vi "Lockin Control Panel.vi"() -> ()   [LabVIEW 2021]
uses:
  <instrlib>/Stanford Research 830/Public/Data/Read (All Parameters).vi
  <instrlib>/Stanford Research 830/Stanford Research 830.lvlib
panel:
  in  "Display 2 Sel":u16(ring)=1 items=["X", "Y", "R", "Theta", "Aux In 1", "Aux In 2", "Aux In 3", "Aux In 4", "Ref Freq", "Ch1 Disp", "Ch2 Disp"]
  in  "Display 1 Sel":u16(ring)=1 items=["X", "Y", "R", "Theta", "Aux In 1", "Aux In 2", "Aux In 3", "Aux In 4", "Ref Freq", "Ch1 Disp", "Ch2 Disp"]
  out "Display 2":dbl format="%.3p"
  in  "Update":bool
  out "Display 1":dbl format="%.3p"
  in  "Reset":bool
  in  "Init":bool
  in  "Set Input":bool
  in  "Float/GND":bool
  in  "AC/DC":bool
  in  "Input":u16(ring) items=["A", "A-B", "I (1MOhm", "I (100MOhm"]
  in  "Refresh":bool
  in  "Auto Phase":bool
  in  "Set Ref":bool
  in  "Phase":dbl
  in  "Reference Source":u16(ring) items=["External", "Internal"]
  in  "Time Constant":u16(ring) items=["10 us", "30 us", "100 us", "300 us", "1 ms", "3 ms", "10 ms", "30 ms", "100 ms", "300 ms", "1 s", "3 s", "10 s", "30 s", "100 s", "300 s", "1 ks", "3 ks", "10 ks", "30 ks"]
  in  "Set TC and SEN":bool
  in  "Sensitivity":i16(ring)=-1 items=["2 nV/fA", "5 nV/fA", "10 nV/fA", "20 nV/fA", "50 nV/fA", "100 nV/fA", "200 nV/fA", "500 nV/fA", "1 uV/pA", "2 uV/pA", "5 uV/pA", "10 uV/pA", "20 uV/pA", "50 uV/pA", "100 uV/pA", "200 uV/pA", "500 uV/pA", "1 mV/nA", "2 mV/nA", "5 mV/nA", "10 mV/nA", "20 mV/nA", "50 mV/nA", "100 mV/nA", "200 mV/nA", "500 mV/nA", "1 V/uA"]
  in  "Quit":bool
  in  "Set OSC":bool
  in  "Amplitude":dbl format="%.6f V"
  in  "Frequency":dbl format="%.3f Hz"
  in  "Connect":bool
  in  "Model":enum16{"7265", "SR830"}(ring)=enum."SR830"
  in  "VISA resource name":refnum<visa-resource-name>
  # "Input"
  # "Measure"
  # "Reference"
  # "Oscillator"
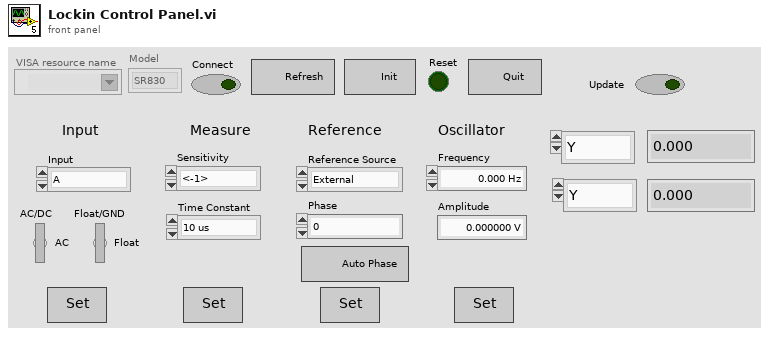
[diagram p1: front panel]
types:
  T1 = enum8{"Enabled", "Disabled", "Disabled and Grayed Out"}
  T2 = cluster{"X-Value":dbl, "Y-Value":dbl, "R-Value":dbl, "Theta-Value":dbl, "Aux In 1 Value":dbl, "Aux In 2 Value":dbl, "Aux In 3 Value":dbl, "Aux In 4 Value":dbl, "Reference Frequency":dbl, "Channel 1 Display":dbl, "Channel 2 Display":dbl}
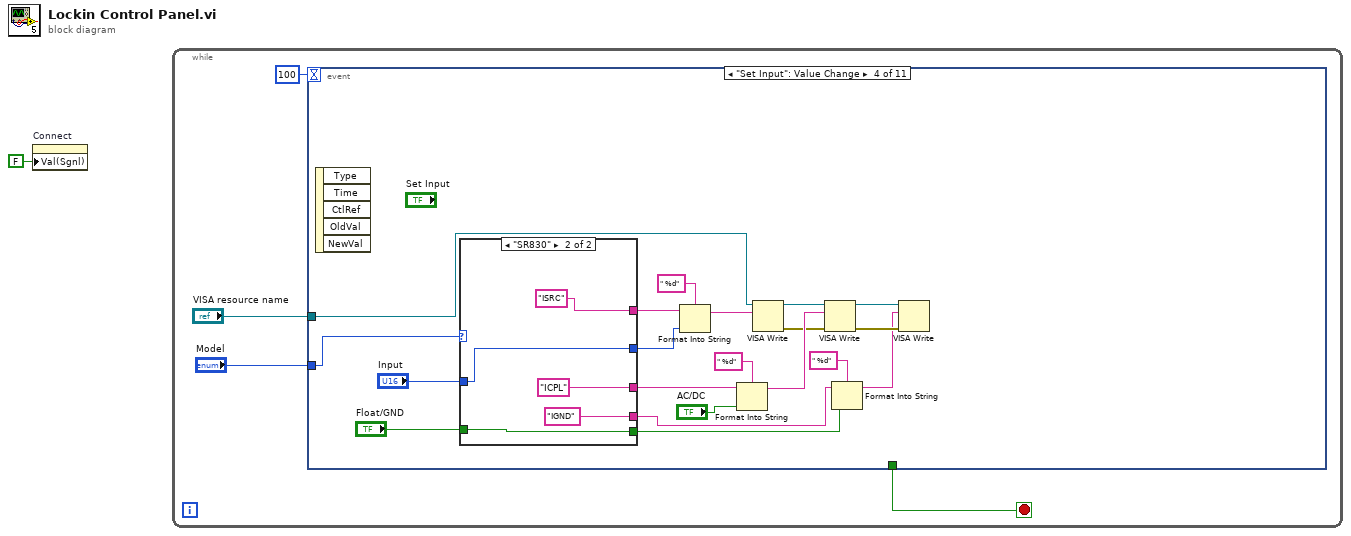
[diagram p0: block diagram]
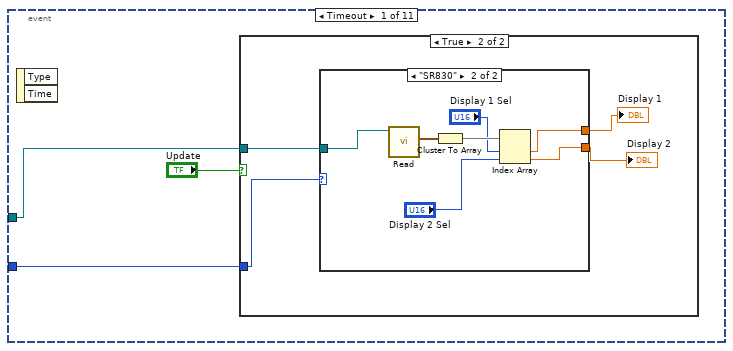
[diagram p2: hidden frame]
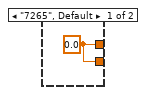
[diagram p4: hidden frame]
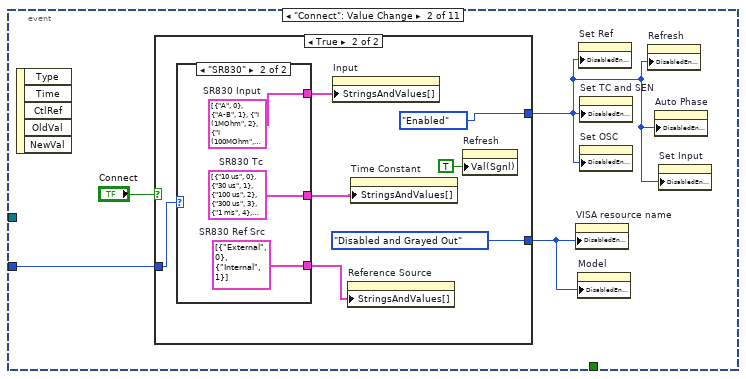
[diagram p5: hidden frame]
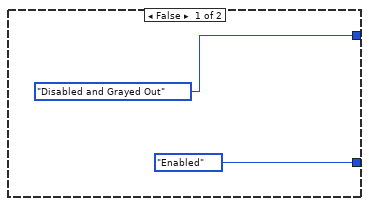
[diagram p6: hidden frame]
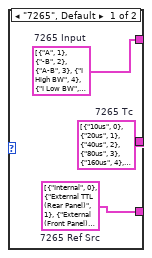
[diagram p7: hidden frame]
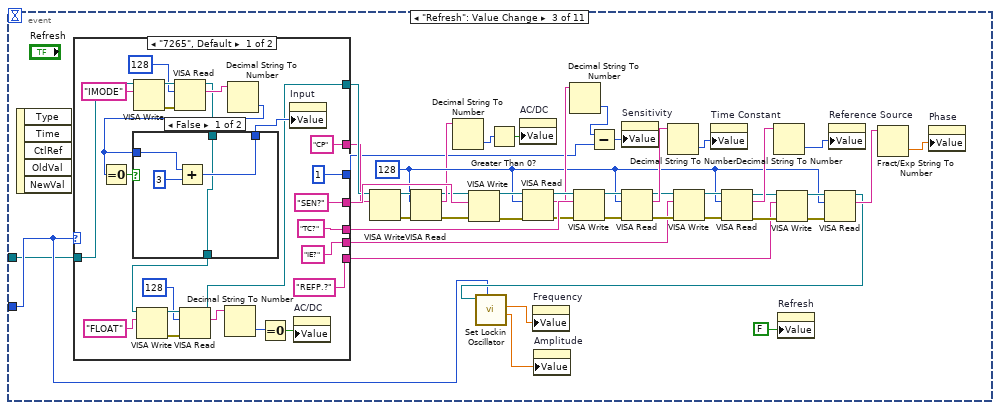
[diagram p8: hidden frame]
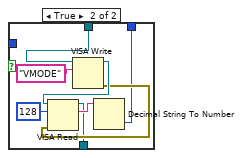
[diagram p9: hidden frame]
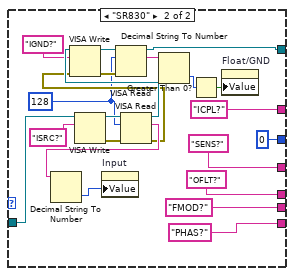
[diagram p10: hidden frame]
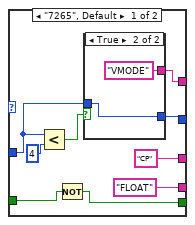
[diagram p11: hidden frame]
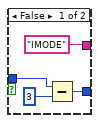
[diagram p12: hidden frame]
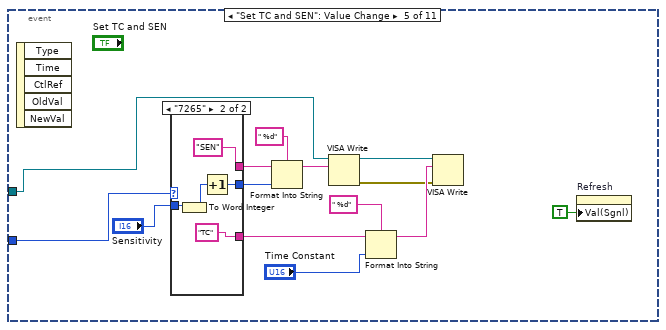
[diagram p13: hidden frame]
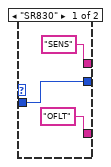
[diagram p14: hidden frame]
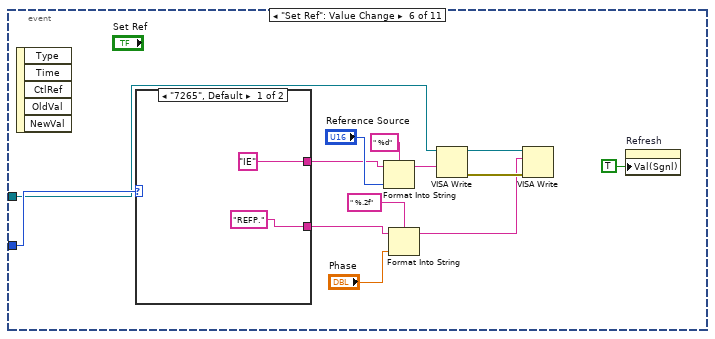
[diagram p15: hidden frame]
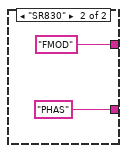
[diagram p16: hidden frame]
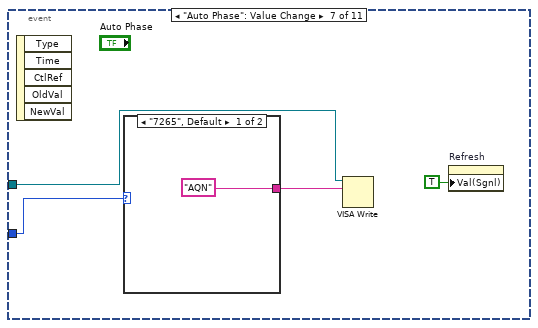
[diagram p17: hidden frame]
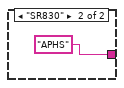
[diagram p18: hidden frame]
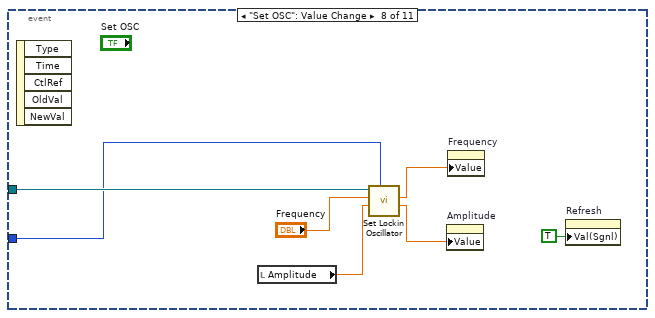
[diagram p19: hidden frame]
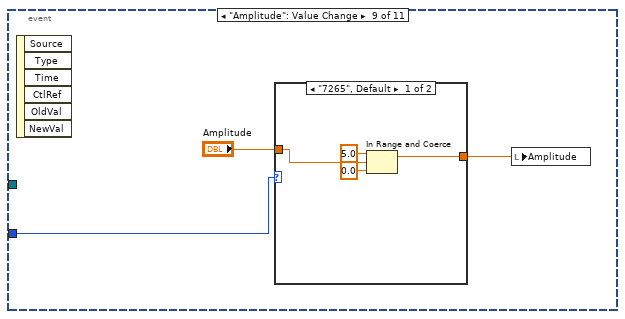
[diagram p20: hidden frame]
diagram:
  n1 = property on="Connect" class="Bool (strict)"("Val(Sgnl)"=FALSE ("Value (Signaling)")) -> ()  [unwired: 2 in, 2 out]
  n2 = while {
    stop <- w5 stop-if-true
    n3 = event shown="[3] \"Set Input\": Value Change" {
      selector: _ -> [_ _ _ _ _ _ _ _ _ _ _]
      dyn-events: _ -> [_ _ _ _ _ _ _ _ _ _ _]
      timeout: 100 -> [_ _ _ _ _ _ _ _ _ _ _]
      tunnel: [_ _ _ _ _ _ _ _ _ _ "Quit"] -> w5
      tunnel: "VISA resource name" -> [w7 _ w50 w156 w196 w213 w223 w234 _ w246 _]
      tunnel: "Model" -> [w6 w23 w58 w162 w195 w217 w225 w233 w237 w247 _]
      event Timeout {
        n4 = event-data() -> ()  [unwired: 1 in, 2 out]
        n5 = case shown="True" "Update" {
          tunnel: w7 -> [_ w12]
          tunnel: w6 -> [_ w11]
          frame False {
          }
          frame True {
            n6 = case shown="\"SR830\"" w11 {
              tunnel: w12 -> [_ w20]
              tunnel: [w13 w16] -> w10
              tunnel: [w13 w15] -> w9
              frame "7265", Default {
                w13 = 0.0 ("X-Value")
              }
              frame "SR830" {
                n7 = call-poly <instrlib>:"Read.vi"("VISA resource name"=w20) -> ("Parameter Values"=w19:T2)  [unwired: 8 in, 2 out]
                n8 = Cluster To Array(cluster=w19) -> (array=w18:dbl[])
                n9 = Index Array(array=w18, index #1="Display 1 Sel", index #2="Display 2 Sel") -> (element #1=w16:dbl, element #2=w15:dbl)
              }
            }
            "Display 1" <- w10
            "Display 2" <- w9
          }
        }
      }
      event "Connect": Value Change {
        n10 = event-data() -> ()  [unwired: 1 in, 5 out]
        n11 = case shown="True" "Connect" {
          tunnel: w23 -> [_ w33]
          tunnel: [T1."Enabled" ("Disabled") T1."Disabled and Grayed Out" ("Disabled")] -> w22
          tunnel: [T1."Disabled and Grayed Out" ("Disabled") T1."Enabled" ("Disabled")] -> w21
          frame False {
          }
          frame True {
            n12 = case shown="\"SR830\"" w33 {
              tunnel: [w36 w39] -> w32
              tunnel: [w35 w38] -> w29
              tunnel: [w34 w37] -> w27
              frame "7265", Default {
                w34 = cluster{"String":string, "Value":u16}[] [{"String"="A", "Value"=1}, {"String"="-B", "Value"=2}, {"String"="A-B", "Value"=3}, {"String"="I High BW", "Value"=4}, {"String"="I Low BW", "Value"=5}]  # 7265 Input
                w35 = cluster{"String":string, "Value":u8}[] [{"String"="Internal", "Value"=0}, {"String"="External TTL (Rear Panel)", "Value"=1}, {"String"="External (Front Panel)", "Value"=2}]  # 7265 Ref Src
                w36 = cluster{"String":string, "Value":u16}[] [{"String"="10us", "Value"=0}, {"String"="20us", "Value"=1}, {"String"="40us", "Value"=2}, {"String"="80us", "Value"=3}, {"String"="160us", "Value"=4}, {"String"="320us", "Value"=5}, {"String"="640us", "Value"=6}, {"String"="5ms", "Value"=7}, {"String"="10ms", "Value"=8}, {"String"="20ms", "Value"=9}, {"String"="50ms", "Value"=10}, {"String"="100ms", "Value"=11}, {"String"="200ms", "Value"=12}, {"String"="500ms", "Value"=13}, {"String"="1s", "Value"=14}, {"String"="2s", "Value"=15}, {"String"="5s", "Value"=16}, {"String"="10s", "Value"=17}, {"String"="20s", "Value"=18}, {"String"="50s", "Value"=19}, {"String"="100s", "Value"=20}, {"String"="200s", "Value"=21}, {"String"="500s", "Value"=22}, {"String"="1ks", "Value"=23}, {"String"="2ks", "Value"=24}, {"String"="5ks", "Value"=25}, {"String"="10ks", "Value"=26}, {"String"="20ks", "Value"=27}, {"String"="50ks", "Value"=28}, {"String"="100ks", "Value"=29}]  # 7265 Tc
              }
              frame "SR830" {
                w37 = cluster{"String":string, "Value":u16}[] [{"String"="A", "Value"=0}, {"String"="A-B", "Value"=1}, {"String"="I (1MOhm", "Value"=2}, {"String"="I (100MOhm", "Value"=3}]  # SR830 Input
                w38 = cluster{"String":string, "Value":u16}[] [{"String"="External", "Value"=0}, {"String"="Internal", "Value"=1}]  # SR830 Ref Src
                w39 = cluster{"String":string, "Value":u16}[] [{"String"="10 us", "Value"=0}, {"String"="30 us", "Value"=1}, {"String"="100 us", "Value"=2}, {"String"="300 us", "Value"=3}, {"String"="1 ms", "Value"=4}, {"String"="3 ms", "Value"=5}, {"String"="10 ms", "Value"=6}, {"String"="30 ms", "Value"=7}, {"String"="100 ms", "Value"=8}, {"String"="300 ms", "Value"=9}, {"String"="1 s", "Value"=10}, {"String"="3 s", "Value"=11}, {"String"="10 s", "Value"=12}, {"String"="30 s", "Value"=13}, {"String"="100 s", "Value"=14}, {"String"="300 s", "Value"=15}, {"String"="1 ks", "Value"=16}, {"String"="3 ks", "Value"=17}, {"String"="10 ks", "Value"=18}, {"String"="30 ks", "Value"=19}]  # SR830 Tc
              }
            }
            n13 = property on="Input" class="Ring (strict)"("StringsAndValues[]"=w27) -> ()  [unwired: 2 in, 2 out]
            n14 = property on="Reference Source" class="Ring (strict)"("StringsAndValues[]"=w29) -> ()  [unwired: 2 in, 2 out]
            n15 = property on="Time Constant" class="Ring (strict)"("StringsAndValues[]"=w32) -> ()  [unwired: 2 in, 2 out]
            n16 = property on="Refresh" class="Bool (strict)"("Val(Sgnl)"=TRUE ("Value (Signaling)")) -> ()  [unwired: 2 in, 2 out]
          }
        }
        n17 = property on="VISA resource name" class="VISAName"("DisabledEnum"=w22) -> ()  [unwired: 2 in, 2 out]
        n18 = property on="Model" class="Enum (strict)"("DisabledEnum"=w22) -> ()  [unwired: 2 in, 2 out]
        n19 = property on="Set Ref" class="Bool"("DisabledEnum"=w21) -> ()  [unwired: 2 in, 2 out]
        n20 = property on="Set TC and SEN" class="Bool"("DisabledEnum"=w21) -> ()  [unwired: 2 in, 2 out]
        n21 = property on="Set OSC" class="Bool"("DisabledEnum"=w21) -> ()  [unwired: 2 in, 2 out]
        n22 = property on="Refresh" class="Bool (strict)"("DisabledEnum"=w21) -> ()  [unwired: 2 in, 2 out]
        n23 = property on="Auto Phase" class="Bool"("DisabledEnum"=w21) -> ()  [unwired: 2 in, 2 out]
        n24 = property on="Set Input" class="Bool"("DisabledEnum"=w21) -> ()  [unwired: 2 in, 2 out]
      }
      event "Refresh": Value Change {
        w48 = u32 128 ("byte count")
        n25 = event-data() -> ()  [unwired: 1 in, 5 out]
        n26 = case shown="\"7265\", Default" w58 {
          tunnel: ["SEN?" "SENS?"] -> w49
          tunnel: ["TC?" "OFLT?"] -> w81
          tunnel: ["IE?" "FMOD?"] -> w69
          tunnel: ["REFP.?" "PHAS?"] -> w62
          tunnel: ["CP" "ICPL?"] -> w43
          tunnel: w50 -> [w103 w134]
          tunnel: [w87 w123] -> w46
          tunnel: [1 0] -> w40
          frame "7265", Default {
            n27 = VISA Write(VISA resource name=w103, write buffer="IMODE") -> (VISA resource name out=w102:refnum<visa-resource-name>, error out=w100:errorcluster)  [unwired: 1 in, 1 out]
            n28 = VISA Read(VISA resource name=w102, byte count=128, error in (no error)=w100) -> (VISA resource name out=w95:refnum<visa-resource-name>, read buffer=w98:string)  [unwired: 2 out]
            n29 = Decimal String To Number(string=w98) -> (number=w96:i32)  [unwired: 2 in, 1 out]
            n30 = Equal To 0?(x=w96) -> (x = 0?=w97:bool)
            n31 = case shown="False" w97 {
              tunnel: w96 -> [w112 _]
              tunnel: w95 -> [w109 w120]
              tunnel: [w110 w114] -> w94
              tunnel: [w109 w113] -> w92
              frame False {
                n32 = Add(x=w112, y=3) -> (x+y=w110:i32)
              }
              frame True {
                n33 = VISA Write(VISA resource name=w120, write buffer="VMODE") -> (VISA resource name out=w118:refnum<visa-resource-name>, error out=w117:errorcluster)  [unwired: 1 in, 1 out]
                n34 = VISA Read(VISA resource name=w118, byte count=u32 128, error in (no error)=w117) -> (VISA resource name out=w113:refnum<visa-resource-name>, read buffer=w115:string)  [unwired: 2 out]
                n35 = Decimal String To Number(string=w115) -> (number=w114:i32)  [unwired: 2 in, 1 out]
              }
            }
            n36 = VISA Write(VISA resource name=w92, write buffer="FLOAT") -> (VISA resource name out=w91:refnum<visa-resource-name>, error out=w89:errorcluster)  [unwired: 1 in, 1 out]
            n37 = VISA Read(VISA resource name=w91, byte count=u32 128, error in (no error)=w89) -> (VISA resource name out=w87:refnum<visa-resource-name>, read buffer=w88:string)  [unwired: 2 out]
            n38 = Decimal String To Number(string=w88) -> (number=w86:i32)  [unwired: 2 in, 1 out]
            n39 = Equal To 0?(x=w86) -> (x = 0?=w85:bool)
            n40 = property on="Input" class="Ring (strict)"("Value"=w94) -> ()  [unwired: 2 in, 2 out]
            n41 = property on="AC/DC" class="Bool (strict)"("Value"=w85) -> ()  [unwired: 2 in, 2 out]
          }
          frame "SR830" {
            w122 = u32 128 ("byte count")
            n42 = VISA Write(VISA resource name=w134, write buffer="ISRC?") -> (VISA resource name out=w137:refnum<visa-resource-name>, error out=w136:errorcluster)  [unwired: 1 in, 1 out]
            n43 = VISA Read(VISA resource name=w137, byte count=w122, error in (no error)=w136) -> (VISA resource name out=w130:refnum<visa-resource-name>, read buffer=w132:string, error out=w129:errorcluster)  [unwired: 1 out]
            n44 = Decimal String To Number(string=w132) -> (number=w133:i32)  [unwired: 2 in, 1 out]
            n45 = VISA Write(VISA resource name=w130, write buffer="IGND?", error in (no error)=w129) -> (VISA resource name out=w131:refnum<visa-resource-name>, error out=w128:errorcluster)  [unwired: 1 out]
            n46 = property on="Input" class="Ring (strict)"("Value"=w133) -> ()  [unwired: 2 in, 2 out]
            n47 = VISA Read(VISA resource name=w131, byte count=w122, error in (no error)=w128) -> (VISA resource name out=w123:refnum<visa-resource-name>, read buffer=w124:string)  [unwired: 2 out]
            n48 = Decimal String To Number(string=w124) -> (number=w126:i32)  [unwired: 2 in, 1 out]
            n49 = Greater Than 0?(x=w126) -> (x > 0?=w125:bool)
            n50 = property on="Float/GND" class="Bool (strict)"("Value"=w125) -> ()  [unwired: 2 in, 2 out]
          }
        }
        n51 = VISA Write(VISA resource name=w46, write buffer=w43) -> (VISA resource name out=w53:refnum<visa-resource-name>, error out=w54:errorcluster)  [unwired: 1 in, 1 out]
        n52 = VISA Read(VISA resource name=w53, byte count=w48, error in (no error)=w54) -> (VISA resource name out=w44:refnum<visa-resource-name>, read buffer=w47:string, error out=w45:errorcluster)  [unwired: 1 out]
        n53 = Decimal String To Number(string=w47) -> (number=w52:i32)  [unwired: 2 in, 1 out]
        n54 = VISA Write(VISA resource name=w44, write buffer=w49, error in (no error)=w45) -> (VISA resource name out=w83:refnum<visa-resource-name>, error out=w82:errorcluster)  [unwired: 1 out]
        n55 = Greater Than 0?(x=w52) -> (x > 0?=w51:bool)
        n56 = property on="AC/DC" class="Bool (strict)"("Value"=w51) -> ()  [unwired: 2 in, 2 out]
        n57 = VISA Read(VISA resource name=w83, byte count=w48, error in (no error)=w82) -> (VISA resource name out=w79:refnum<visa-resource-name>, read buffer=w78:string, error out=w80:errorcluster)  [unwired: 1 out]
        n58 = Decimal String To Number(string=w78) -> (number=w42:i32)  [unwired: 2 in, 1 out]
        n59 = VISA Write(VISA resource name=w79, write buffer=w81, error in (no error)=w80) -> (VISA resource name out=w77:refnum<visa-resource-name>, error out=w76:errorcluster)  [unwired: 1 out]
        n60 = Subtract(x=w42, y=w40) -> (x-y=w41:i32)
        n61 = property on="Sensitivity" class="Ring (strict)"("Value"=w41) -> ()  [unwired: 2 in, 2 out]
        n62 = VISA Read(VISA resource name=w77, byte count=w48, error in (no error)=w76) -> (VISA resource name out=w71:refnum<visa-resource-name>, read buffer=w74:string, error out=w70:errorcluster)  [unwired: 1 out]
        n63 = Decimal String To Number(string=w74) -> (number=w75:i32)  [unwired: 2 in, 1 out]
        n64 = VISA Write(VISA resource name=w71, write buffer=w69, error in (no error)=w70) -> (VISA resource name out=w73:refnum<visa-resource-name>, error out=w72:errorcluster)  [unwired: 1 out]
        n65 = property on="Time Constant" class="Ring (strict)"("Value"=w75) -> ()  [unwired: 2 in, 2 out]
        n66 = VISA Read(VISA resource name=w73, byte count=w48, error in (no error)=w72) -> (VISA resource name out=w64:refnum<visa-resource-name>, read buffer=w67:string, error out=w63:errorcluster)  [unwired: 1 out]
        n67 = Decimal String To Number(string=w67) -> (number=w68:i32)  [unwired: 2 in, 1 out]
        n68 = VISA Write(VISA resource name=w64, write buffer=w62, error in (no error)=w63) -> (VISA resource name out=w66:refnum<visa-resource-name>, error out=w65:errorcluster)  [unwired: 1 out]
        n69 = property on="Refresh" class="Bool (strict)"("Value"=FALSE ("Refresh")) -> ()  [unwired: 2 in, 2 out]
        n70 = VISA Read(VISA resource name=w66, byte count=w48, error in (no error)=w65) -> (VISA resource name out=w59:refnum<visa-resource-name>, read buffer=w60:string)  [unwired: 2 out]
        n71 = call "Set Lockin Oscillator.vi"("Model"=w58, "VISA resource name"=w59) -> ("Actual Amp"=w56:dbl, "Actual Freq"=w57:dbl)  [unwired: 8 in]
        n72 = property on="Frequency" class="DigNum (strict)"("Value"=w57) -> ()  [unwired: 2 in, 2 out]
        n73 = property on="Amplitude" class="DigNum (strict)"("Value"=w56) -> ()  [unwired: 2 in, 2 out]
        n74 = property on="Reference Source" class="Ring (strict)"("Value"=w68) -> ()  [unwired: 2 in, 2 out]
        n75 = Fract/Exp String To Number(string=w60) -> (number=w61:dbl)  [unwired: 3 in, 1 out]
        n76 = property on="Phase" class="DigNum (strict)"("Value"=w61) -> ()  [unwired: 2 in, 2 out]
      }
      event "Set Input": Value Change {
        n77 = event-data() -> ()  [unwired: 1 in, 5 out]
        n78 = case shown="\"SR830\"" w162 {
          tunnel: "Input" -> [w167 w182]
          tunnel: [w168 w182] -> w160
          tunnel: [w169 "ISRC"] -> w159
          tunnel: ["CP" "ICPL"] -> w153
          tunnel: ["FLOAT" "IGND"] -> w146
          tunnel: "Float/GND" -> [w164 w178]
          tunnel: [w163 w178] -> w144
          frame "7265", Default {
            n79 = Less?(x=w167, y=u16 4) -> (x < y?=w170:bool)
            n80 = Not(x=w164) -> (.not. x?=w163:bool)
            n81 = case shown="True" w170 {
              tunnel: ["IMODE" "VMODE"] -> w169
              tunnel: [w174 w176] -> w168
              tunnel: w167 -> [w173 w176]
              frame False {
                n82 = Subtract(x=w173, y=u16 3) -> (x-y=w174:u16)
              }
              frame True {
              }
            }
          }
          frame "SR830" {
          }
        }
        n83 = Format Into String(format string=" %d", initial string=w159, w160) -> (resulting string=w157:string)  [unwired: 1 in, 1 out]
        n84 = Format Into String(format string=" %d", initial string=w153, "AC/DC") -> (resulting string=w151:string)  [unwired: 1 in, 1 out]
        n85 = VISA Write(VISA resource name=w156, write buffer=w157) -> (VISA resource name out=w150:refnum<visa-resource-name>, error out=w149:errorcluster)  [unwired: 1 in, 1 out]
        n86 = VISA Write(VISA resource name=w150, write buffer=w151, error in (no error)=w149) -> (VISA resource name out=w147:refnum<visa-resource-name>, error out=w148:errorcluster)  [unwired: 1 out]
        n87 = Format Into String(format string=" %d", initial string=w146, w144) -> (resulting string=w143:string)  [unwired: 1 in, 1 out]
        n88 = VISA Write(VISA resource name=w147, write buffer=w143, error in (no error)=w148) -> ()  [unwired: 3 out]
      }
      event "Set TC and SEN": Value Change {
        n89 = event-data() -> ()  [unwired: 1 in, 5 out]
        n90 = case shown="\"7265\"" w195 {
          tunnel: ["SENS" "SEN"] -> w194
          tunnel: "Sensitivity" -> [w198 w202]
          tunnel: [w198 w203] -> w191
          tunnel: ["OFLT" "TC"] -> w189
          frame "SR830" {
          }
          frame "7265" {
            n91 = To Word Integer(number=w202) -> (16bit integer=w201:i16)
            n92 = Increment(x=w201) -> (x+1=w203:i16)
          }
        }
        n93 = Format Into String(format string=" %d", initial string=w194, w191) -> (resulting string=w190:string)  [unwired: 1 in, 1 out]
        n94 = VISA Write(VISA resource name=w196, write buffer=w190) -> (VISA resource name out=w186:refnum<visa-resource-name>, error out=w184:errorcluster)  [unwired: 1 in, 1 out]
        n95 = Format Into String(format string=" %d", initial string=w189, "Time Constant") -> (resulting string=w185:string)  [unwired: 1 in, 1 out]
        n96 = VISA Write(VISA resource name=w186, write buffer=w185, error in (no error)=w184) -> ()  [unwired: 3 out]
        n97 = property on="Refresh" class="Bool (strict)"("Val(Sgnl)"=TRUE ("Value (Signaling)")) -> ()  [unwired: 2 in, 2 out]
      }
      event "Set Ref": Value Change {
        n98 = event-data() -> ()  [unwired: 1 in, 5 out]
        n99 = case shown="\"7265\", Default" w217 {
          tunnel: ["IE" "FMOD"] -> w215
          tunnel: ["REFP." "PHAS"] -> w211
          frame "7265", Default {
          }
          frame "SR830" {
          }
        }
        n100 = Format Into String(format string=" %d", initial string=w215, "Reference Source") -> (resulting string=w212:string)  [unwired: 1 in, 1 out]
        n101 = Format Into String(format string=" %.2f", initial string=w211, "Phase") -> (resulting string=w206:string)  [unwired: 1 in, 1 out]
        n102 = VISA Write(VISA resource name=w213, write buffer=w212) -> (VISA resource name out=w207:refnum<visa-resource-name>, error out=w208:errorcluster)  [unwired: 1 in, 1 out]
        n103 = VISA Write(VISA resource name=w207, write buffer=w206, error in (no error)=w208) -> ()  [unwired: 3 out]
        n104 = property on="Refresh" class="Bool (strict)"("Val(Sgnl)"=TRUE ("Value (Signaling)")) -> ()  [unwired: 2 in, 2 out]
      }
      event "Auto Phase": Value Change {
        n105 = event-data() -> ()  [unwired: 1 in, 5 out]
        n106 = case shown="\"7265\", Default" w225 {
          tunnel: ["AQN" "APHS"] -> w224
          frame "7265", Default {
          }
          frame "SR830" {
          }
        }
        n107 = VISA Write(VISA resource name=w223, write buffer=w224) -> ()  [unwired: 1 in, 3 out]
        n108 = property on="Refresh" class="Bool (strict)"("Val(Sgnl)"=TRUE ("Value (Signaling)")) -> ()  [unwired: 2 in, 2 out]
      }
      event "Set OSC": Value Change {
        n109 = event-data() -> ()  [unwired: 1 in, 5 out]
        n110 = local read "Amplitude"() -> (w228:dbl)
        n111 = call "Set Lockin Oscillator.vi"("Model"=w233, "Amplitude"=w228, "Frequency"="Frequency", "VISA resource name"=w234) -> ("Actual Amp"=w230:dbl, "Actual Freq"=w231:dbl)  [unwired: 6 in]
        n112 = property on="Amplitude" class="DigNum (strict)"("Value"=w230) -> ()  [unwired: 2 in, 2 out]
        n113 = property on="Frequency" class="DigNum (strict)"("Value"=w231) -> ()  [unwired: 2 in, 2 out]
        n114 = property on="Refresh" class="Bool (strict)"("Val(Sgnl)"=TRUE ("Value (Signaling)")) -> ()  [unwired: 2 in, 2 out]
      }
      event "Amplitude": Value Change {
        n115 = event-data() -> ()  [unwired: 1 in, 6 out]
        n116 = case shown="\"7265\", Default" w237 {
          tunnel: "Amplitude" -> [w238 w245]
          tunnel: [w239 w242] -> w235
          frame "7265", Default {
            n117 = In Range and Coerce(upper limit=5.0, x=w238, lower limit=0.0) -> (coerced(x)=w239:dbl)  [unwired: 1 out]
          }
          frame "SR830" {
            n118 = In Range and Coerce(upper limit=5.0, x=w245, lower limit=0.004) -> (coerced(x)=w242:dbl)  [unwired: 1 out]
          }
        }
        n119 = local write "Amplitude"(w235) -> ()
      }
      event "Init": Value Change {
        n120 = event-data() -> ()  [unwired: 1 in, 5 out]
        n121 = case shown="\"SR830\"" w247 {
          tunnel: w246 -> [_ w251]
          frame "7265", Default {
            n122 = One Button Dialog(message="You don't need to do that!", button name ("OK")="Got it...") -> ()  [unwired: 1 out]
          }
          frame "SR830" {
            n123 = call <instrlib>:"Initialize.vi"("Reset (True)"="Reset", "VISA resource name"=w251) -> ()  [unwired: 8 in, 2 out]
          }
        }
      }
      event "Quit": Value Change {
        n124 = event-data() -> ()  [unwired: 1 in, 5 out]
      }
    }
  }
